vi "move_zip_path.vi"(6 "zip_move_directory":path, 8 "error in (no error)":errorcluster, 11 "build_artifact":path) -> (0 "error out":errorcluster, 3 "path":path)   [LabVIEW 2015, in "lv-builder-default.lvlib"]
uses:
  lv-builder-default.lvlib
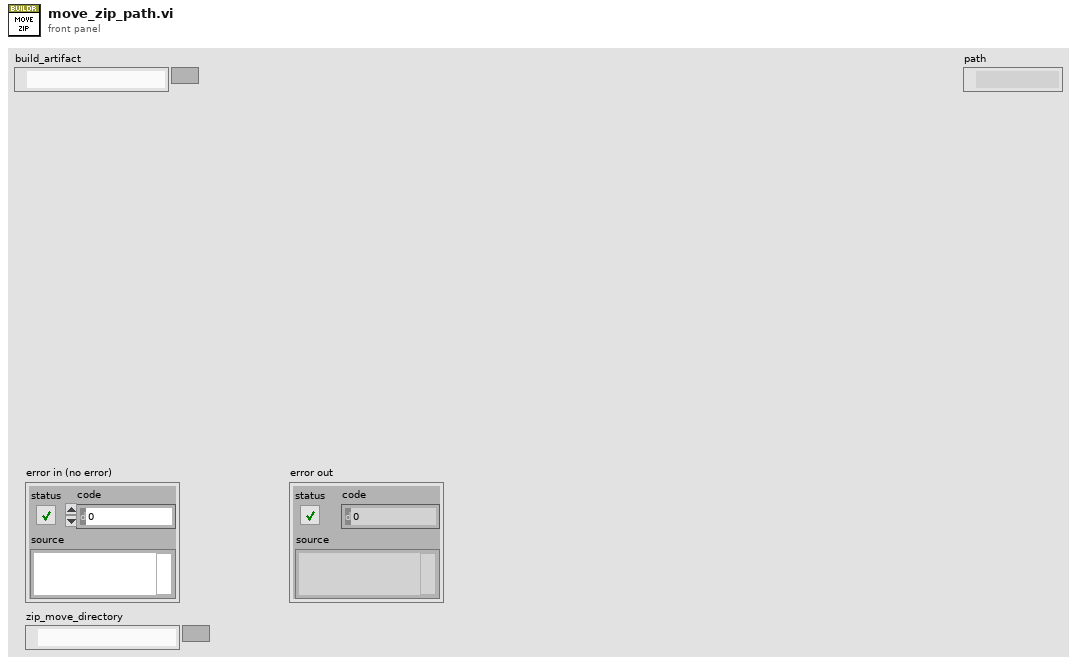
[diagram p1: front panel]
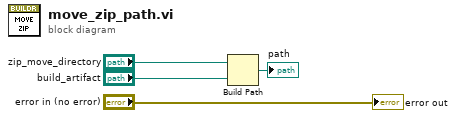
[diagram p0: block diagram]
diagram:
  n1 = Build Path(base path="zip_move_directory", name or relative path="build_artifact") -> (appended path=→"path":path)
  "error out" <- "error in (no error)"
